vi "Tacking Function.vi"() -> ()   [LabVIEW 2011]
uses:
  2x3-RIO-OCU Comm/2x3 Typedefs/ocuWaypoint.ctl
  2x3-RIO-OCU Comm/2x3 Typedefs/waypointTypes.ctl
  2 Typedefs/UTM Location.ctl
  2 Typedefs/Velocity.ctl
  <vilib>/Analysis/coordinate.llb/Absolute Angle Difference (scalar).vi
  <vilib>/Analysis/coordinate.llb/Wrap Angle (scalar).vi
  <vilib>/Analysis/coordinate.llb/Set Angle Unit.vi
  <vilib>/Analysis/NI_AAL_Angle.lvlib
panel:
  out "Jump Length (m)":dbl
  in  "Wind Vector\nScaling Factor":dbl
  out "Intermediate\nWaypoints":T1[](array[typedef]) {"Point Type" items=["Drive", "Round Port", "Round Starboard", "Stay"]}
  out "Tack Waypoint Plot":cluster{"Y":dbl[], "Y":dbl[]}[](graph)
  in  "Minimum Final\nTack Distance (m?)":dbl
  out "Number of jumps":dbl
  out "Angle from boat to waypoint (rad)":dbl
  in  "Bounding box\nside length (m?)":dbl
  out "Wind Direction (green)\nIrons (black)\nMax_angle (blue)\nMin_angle (red)":cluster{dbl, dbl, dbl, dbl}(knob) scale=-3.14..6.28
  # "QUIRK : If the 'Bounding box\nside length is 0 (as on opening)\nthe vi will go into an infinite loop"
  # "Also, you can't see the wind vector\nuntil this scaling factor is non-zero\n(10 - 30 is good)"
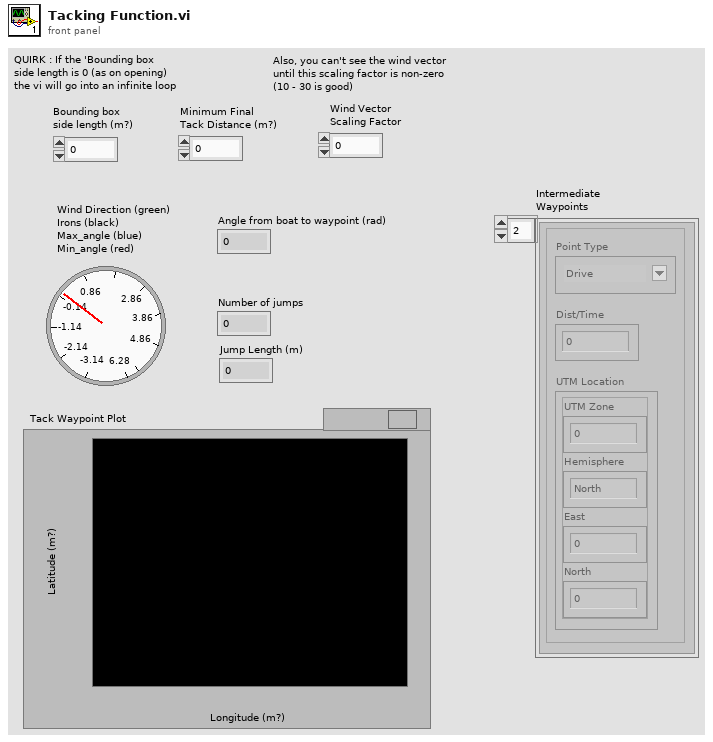
[diagram p1: front panel]
types:
  T1 = typedef "ocuWaypoint.ctl" = cluster{"Point Type":T2, "Dist/Time":dbl, "UTM Location":T3}
  T2 = typedef "waypointTypes.ctl" = u16
  T3 = typedef "UTM Location.ctl" = cluster{"UTM Zone":dbl, "Hemisphere":enum16{"North", "South"}, "East":dbl, "North":dbl}
  T4 = typedef "Velocity.ctl" = cluster{"East":dbl, "North":dbl}
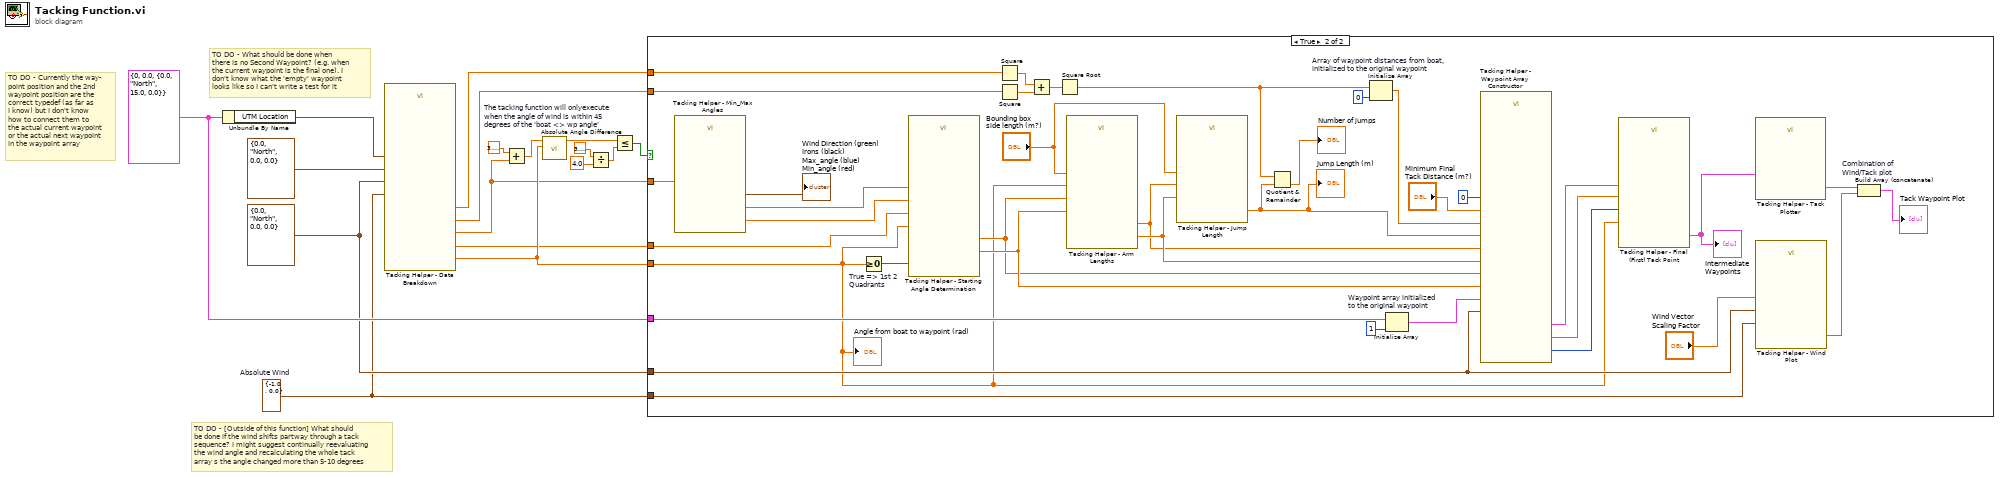
[diagram p0: block diagram]
diagram:
  w1 = T4 {"East"=-1.0, "North"=0.0}  # Absolute Wind
  w3 = T3 {"UTM Zone"=0.0, "Hemisphere"=enum."North", "East"=0.0, "North"=0.0} ("Robot UTM Location")
  w4 = T1 {"Point Type"=0, "Dist/Time"=0.0, "UTM Location"={"UTM Zone"=0.0, "Hemisphere"=enum."North", "East"=15.0, "North"=0.0}} ("Waypoint")
  # "TO DO - Currently the way-\npoint position and the 2nd\nwaypoint position are the\ncorrect typedef (as far as\nI know) but I don't know\nhow to connect them to\nthe actual current waypoint\nor the actual next waypoint\nin the waypoint array"
  # "TO DO - [Outside of this function] What should\nbe done if the wind shifts partway through a tack\nsequence? I might suggest continually reevaluating\nthe wind angle and recalculating the whole tack\narray s the angle changed more than 5-10 degrees"
  # "TO DO - What should be done when\nthere is no Second Waypoint? (e.g. when\nthe current waypoint is the final one). I\ndon't know what the 'empty' waypoint\nlooks like so I can't write a test for it"
  n1 = Unbundle By Name(w4) -> ("UTM Location"=w8:T3)
  n2 = call "Tacking Helper - Data Breakdown.vi"("Absolute\nWind Vector"=w1, "Second\nWaypoint\nPosition"=T3 {"UTM Zone"=0.0, "Hemisphere"=enum."North", "East"=0.0, "North"=0.0} ("UTM Location"), "Boat\nPosition"=w3, "Waypoint\nPosition"=w8) -> ("Angle of Wind"=w10:dbl, "X, boat > wp"=w6:dbl, "Y, boat >wp"=w5:dbl, "Boat <> 2nd wp Angle"=w7:dbl, "Boat <> wp Angle"=w17:dbl)  [unwired: 3 in]
  n3 = Add(x=3.141592653589793, y=w10) -> (x+y=w16:dbl)
  n4 = call-poly <vilib>:"Absolute Angle Difference.vi"("angle 2"=w17, "angle 1"=w16) -> ("absolute angle difference"=w15:dbl)  [unwired: 8 in, 1 out]
  n5 = Divide(x=3.141592653589793, y=4.0) -> (x/y=w12:dbl)
  n6 = Less Or Equal? "The tacking function will onlyexecute\nwhen the angle of wind is within 45\ndegrees of the 'boat <> wp angle'"(x=w15, y=w12) -> (x <= y?=w11:bool)
  n7 = case shown="True" w11 {
    tunnel: w7 -> [_ w18]
    tunnel: w6 -> [_ w53]
    tunnel: w5 -> [_ w52]
    tunnel: w4 -> [_ w47]
    tunnel: w10 -> [_ w45]
    tunnel: w17 -> [_ w19]
    tunnel: w3 -> [_ w32]
    tunnel: w1 -> [_ w34]
    frame False {
    }
    frame True {
      n8 = call "Tacking Helper - Min_Max Angles.vi"("Wind Direction (rad)"=w45) -> ("Irons/Tack\nIndicator"=→"Wind Direction (green)\nIrons (black)\nMax_angle (blue)\nMin_angle (red)":cluster{dbl, dbl, dbl, dbl}, "Max Angle\nof Tack"=w29:dbl, "Min Angle\nof Tack"=w28:dbl)  [unwired: 8 in]
      n9 = Greater Or Equal To 0? "True => 1st 2\nQuadrants"(x=w19) -> (x >= 0?=w44:bool)
      n10 = call "Tacking Helper - Starting Angle Determination.vi"("Boat <> 2nd wp Angle"=w18, "Is the boat to wp\nangle greater than 0?"=w44, "Max Angle\nof Tack"=w29, "Min Angle\nof Tack"=w28, "Angle from boat to waypoint"=w19) -> ("Second Angle"=w42:dbl, "Starting Angle"=w27:dbl)  [unwired: 5 in]
      n11 = Square(x=w53) -> (x^2=w51:dbl)
      n12 = Square(x=w52) -> (x^2=w50:dbl)
      n13 = Add(x=w51, y=w50) -> (x+y=w49:dbl)
      n14 = Square Root(x=w49) -> (sqrt(x)=w33:dbl)
      n15 = call "Tacking Helper - Arm Lengths.vi"("Bounding box\nside length (m?)"="Bounding box\nside length (m?)", "Second Angle"=w42, "Starting Angle"=w27, "Angle from boat\nto waypoint"=w19) -> ("Second\nArm Length"=w43:dbl, "Starting\nArm Length"=w23:dbl)  [unwired: 6 in]
      n16 = call "Tacking Helper - Jump Length.vi"("Bounding box\nside length (m?)"="Bounding box\nside length (m?)", "Second\nArm Length"=w43, "Starting\nArm Length"=w23) -> ("Jump Length (m)"=w24:dbl)  [unwired: 8 in]
      "Jump Length (m)" <- w24
      n17 = Quotient & Remainder(x=w33, y=w24) -> (floor(x/y)=→"Number of jumps":dbl)  [unwired: 1 out]
      n18 = Initialize Array "Array of waypoint distances from boat,\ninitialized to the original waypoint"(w33, 0 ("dimension size")) -> (w39:dbl[])
      n19 = Initialize Array "Waypoint array initialized\nto the original waypoint"(w47, 1 ("dimension size")) -> (w41:T1[])
      n20 = call "Tacking Helper - Waypoint Array Constructor.vi"("Second Angle"=w42, "Minimum Final Tack Distance (m?)"="Minimum Final\nTack Distance (m?)", "Starting\nArm Length"=w23, "Second\nArm Length"=w43, "Jump Length (m)"=w24, "Starting Angle"=w27, "Distance of each waypoint to boat"=w39, "Array Beginning"=0, "Waypoint Array In"=w41, "Boat Position"=w32) -> ("Distance to boat"=w25:dbl, "Final Index of\nWaypoint Array"=w38:i32, "Intermediate \nWaypoint Array out"=w22:T1[])  [unwired: 3 in]
      n21 = call "Tacking Helper - Final (First) Tack Point.vi"("Intermediate\nWaypoints In"=w22, "Angle from boat to waypoint"=w19, "End of Array"=w38, "Distance to boat"=w25) -> ("Intermediate\nWaypoints Out"=w37:T1[])  [unwired: 7 in]
      "Intermediate\nWaypoints" <- w37
      n22 = call "Tacking Helper - Tack Plotter.vi"("Intermediate\nWaypoints In"=w37) -> ("Tack Plot Data Out"=w36:cluster{dbl[], dbl[]}[])  [unwired: 10 in]
      n23 = call "Tacking Helper - Wind Plot.vi"("Boat\nPosition"=w32, "Wind Vector\nTop = x\nBottom = y"=w34, "Wind Vector\nScaling Factor"="Wind Vector\nScaling Factor") -> ("Output Cluster\nFor Plotting"=w30:cluster{dbl[], dbl[]})  [unwired: 8 in]
      n24 = Build Array (concatenate) "Combination of\nWind/Tack plot"(w36, w30) -> (→"Tack Waypoint Plot":cluster{dbl[], dbl[]}[])
      "Angle from boat to waypoint (rad)" <- w19
    }
  }
